vi "Write Error to System Log.vi"(6 "log each error instance (F)":bool, 8 "error in":errorcluster, 11 "identifier":string) -> (0 "error out":errorcluster)   [LabVIEW 2024, in "AIM ARINC 429 Engine.lvlib" / "Custom Device.lvlib"]
uses:
  Custom Device.lvlib
  ca55ed61-c1f5-4d13-8aef-490b87d2cf89.vi
  <vilib>/NI VeriStand/Custom Device Tools/Custom Device Utility Library/Custom Device Utility Library.lvlib
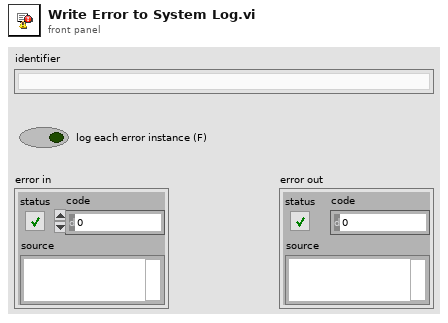
[diagram p1: front panel]
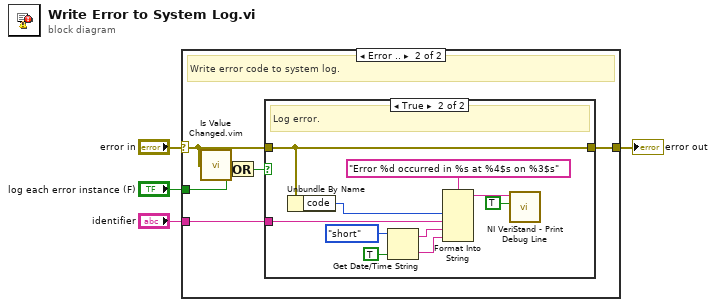
[diagram p0: block diagram]
diagram:
  n1 = case shown="Error .." "error in" {
    selector: "error in" -> [w5 w10]
    tunnel: [w5 w11] -> w4
    tunnel: "log each error instance (F)" -> [_ w7]
    tunnel: "identifier" -> [_ w6]
    frame No Error {
      # "Do not log OK - this is not a heartbeat.\nDo not log warnings."
    }
    frame Error {
      # "Write error code to system log."
      n2 = call "Is Value Changed.vim"("value"=w10) -> ("changed or first call?"=w8:bool)
      n3 = Or(x=w8, y=w7) -> (x .or. y?=w9:bool)
      n4 = case shown="True" w9 {
        tunnel: w10 -> [w12 w14]
        tunnel: [w12 w14] -> w11
        tunnel: w6 -> [_ w13]
        frame False {
          # "Do not log error."
        }
        frame True {
          # "Log error."
          n5 = Unbundle By Name(w14) -> ("code"=w22:i32)
          n6 = Get Date/Time String(date format (0)=enum16{"short", "long", "abbreviated"}."short", want seconds? (F)=TRUE) -> (date string=w19:string, time string=w18:string)  [unwired: 1 in]
          n7 = Format Into String(format string="Error %d occurred in %s at %4$s on %3$s", w22, w13, w19, w18) -> (resulting string=w20:string)  [unwired: 2 in, 1 out]
          n8 = call <vilib>:"NI VeriStand - Print Debug Line.vi"("Add to log file? (F)"=TRUE, "Message"=w20) -> ()  [unwired: 9 in, 1 out]
        }
      }
    }
  }
  "error out" <- w4
